vi "Verify empty array.vi"(11 "Entradas":string[](array[string])) -> (3 "Is Null?":bool)   [LabVIEW 2018]
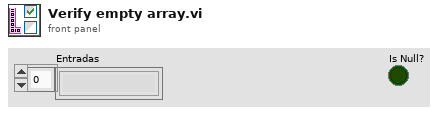
[diagram p1: front panel]
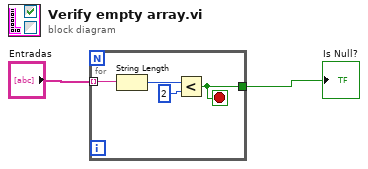
[diagram p0: block diagram]
diagram:
  n1 = for {
    tunnel: "Entradas" -> [w6] mode=indexing
    tunnel: [w3] -> w1
    stop <- w3 stop-if-true
    n2 = String Length(string=w6) -> (length=w5:i32)
    n3 = Less?(x=w5, y=2) -> (x < y?=w3:bool)
  }
  "Is Null?" <- w1
